vi "Close_Actor_Test.vi"(8 "error in (no error)":errorcluster caption="entrée d'erreur (pas d'erreur)", 11 "Test (Default) en entrée":refnum<class "Actor Test (Default).lvclass">) -> (0 "error out":errorcluster caption="sortie d'erreur", 3 "Test (Default) en sortie":refnum<class "Actor Test (Default).lvclass">)   [LabVIEW 2020, in "Library Core.lvlib" / "Actor Test (Default).lvclass"]
uses:
  Actor Test (Default).lvclass
  Actor Test (Default).lvclass/Actor Test (Default).ctl
  Commun VI/Library Commun.lvlib
panel:
  out "Time of Test":u32
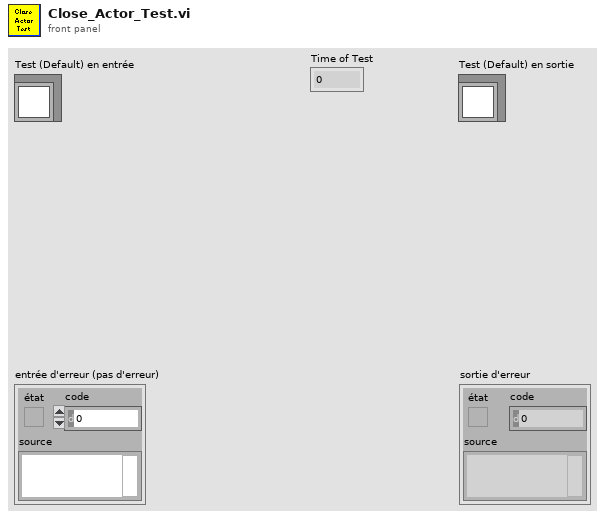
[diagram p1: front panel]
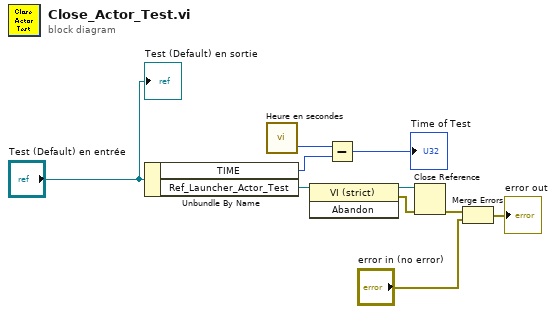
[diagram p0: block diagram]
diagram:
  n1 = Unbundle By Name("Test (Default) en entrée") -> ("TIME"=w5:u32, "Ref_Launcher_Actor_Test"=w6:refnum<vi>)
  n2 = call "Heure en secondes.vi"() -> ("Heure en milisecondes"=w4:u32)  [unwired: 2 in, 1 out]
  n3 = invoke class="VI (strict)" method="Abandon"(reference=w6) -> (reference out=w2:refnum<vi>, error out=w1:errorcluster)  [unwired: 2 in, 1 out]
  n4 = Subtract(x=w4, y=w5) -> (x-y=→"Time of Test":u32)
  n5 = Close Reference(reference=w2, error in (no error)=w1) -> (error out=w9:errorcluster)
  n6 = Merge Errors(w9, "error in (no error)") -> (→"error out":errorcluster)
  "Test (Default) en sortie" <- "Test (Default) en entrée"
